vi "Plot menu activation location.vi"(8 "error in (no error)":errorcluster, 11 "MenuRef":refnum<k9>) -> (0 "error out":errorcluster, 1 "submenu tags":string[](array[string]), 2 "Location":T1, 3 "menu reference out":refnum<k9>)   [LabVIEW 2021, in "RocketPlot.lvlib"]
uses:
  RocketPlot.lvlib
  Plot menu activation submenu type.ctl
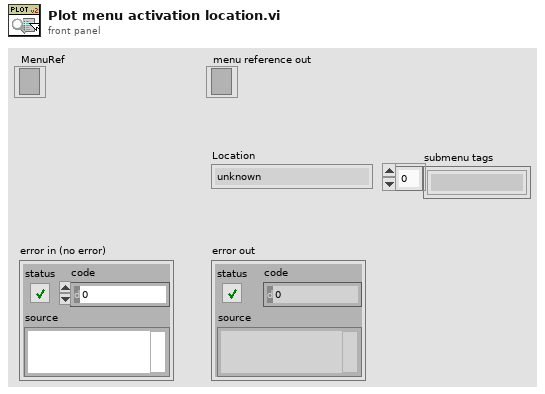
[diagram p1: front panel]
types:
  T1 = typedef "RocketPlot.lvlib/Plot menu activation submenu type.ctl" = enum16{"unknown", "plot", "legend", "x-markers", "x-scale", "y-markers", "y-scale"}
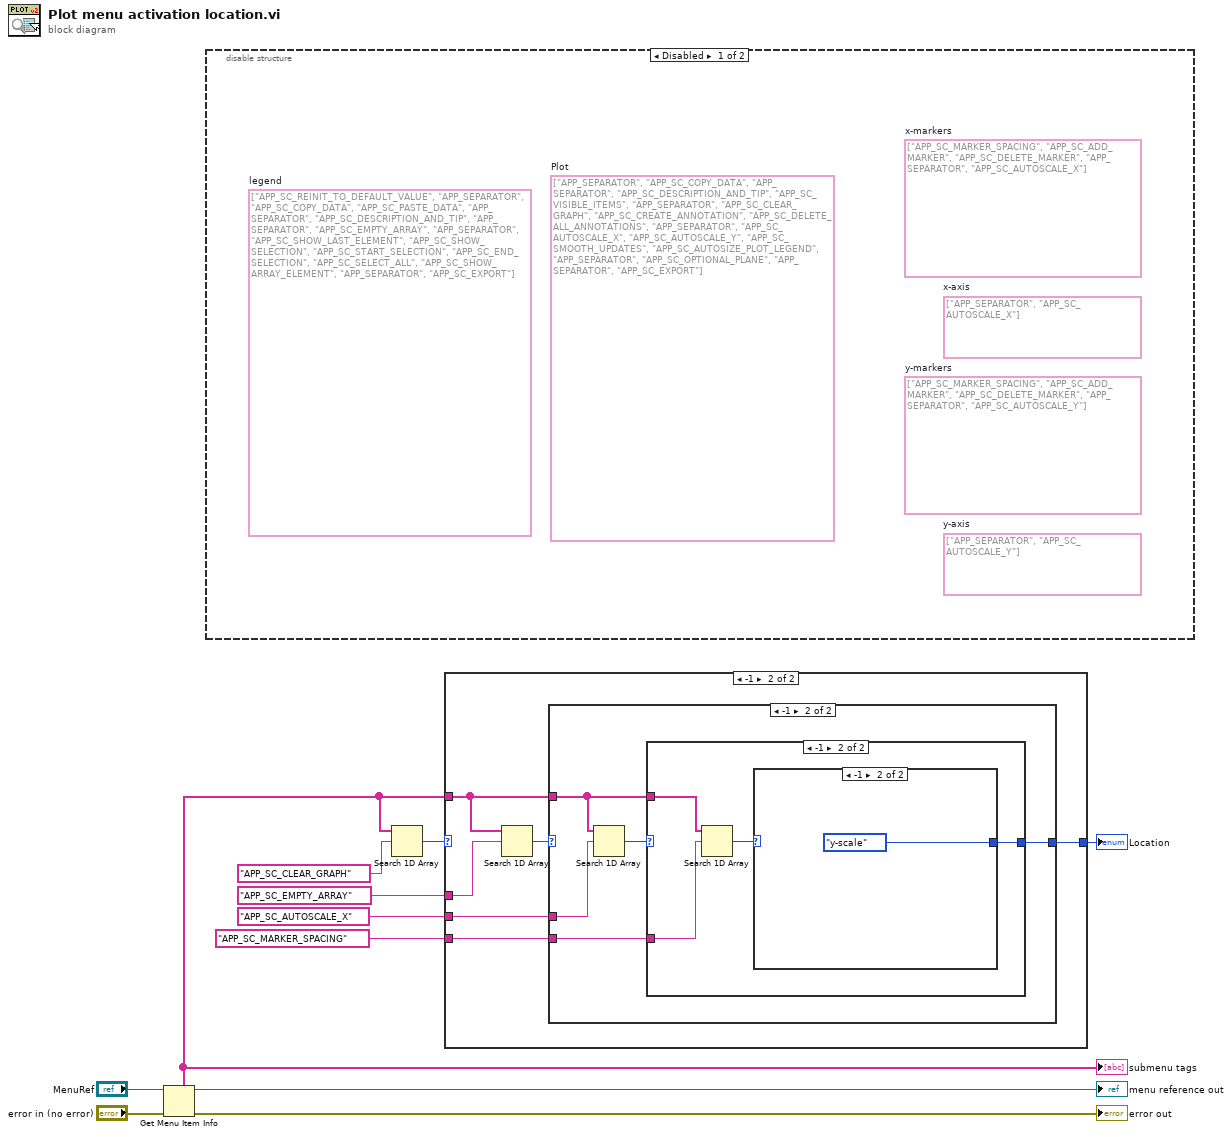
[diagram p0: block diagram]
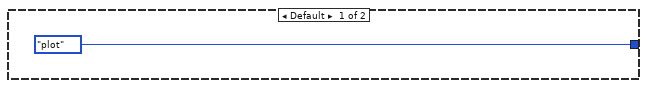
[diagram p3: hidden frame]
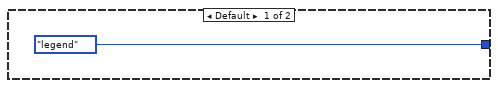
[diagram p4: hidden frame]
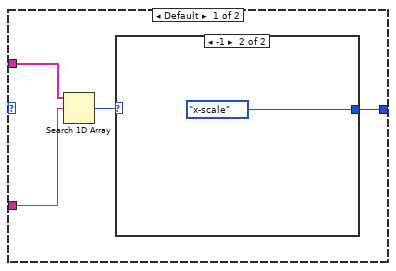
[diagram p5: hidden frame]
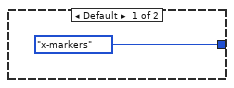
[diagram p6: hidden frame]
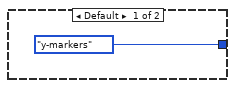
[diagram p7: hidden frame]
diagram:
  n1 = Get Menu Item Info(8:"error in (no error)", 11:"MenuRef") -> (0:→"error out":errorcluster, 3:→"menu reference out":refnum<k9>, 5:w5:string[])  [unwired: 1 in, 4 out]
  "submenu tags" <- w5
  n2 = disable-structure shown="Disabled" {
    frame Disabled {
      (unwired) string[] ["APP_SC_REINIT_TO_DEFAULT_VALUE", "APP_SEPARATOR", "APP_SC_COPY_DATA", "APP_SC_PASTE_DATA", "APP_SEPARATOR", "APP_SC_DESCRIPTION_AND_TIP", "APP_SEPARATOR", "APP_SC_EMPTY_ARRAY", "APP_SEPARATOR", "APP_SC_SHOW_LAST_ELEMENT", "APP_SC_SHOW_SELECTION", "APP_SC_START_SELECTION", "APP_SC_END_SELECTION", "APP_SC_SELECT_ALL", "APP_SC_SHOW_ARRAY_ELEMENT", "APP_SEPARATOR", "APP_SC_EXPORT"]  # legend
      (unwired) string[] ["APP_SEPARATOR", "APP_SC_COPY_DATA", "APP_SEPARATOR", "APP_SC_DESCRIPTION_AND_TIP", "APP_SC_VISIBLE_ITEMS", "APP_SEPARATOR", "APP_SC_CLEAR_GRAPH", "APP_SC_CREATE_ANNOTATION", "APP_SC_DELETE_ALL_ANNOTATIONS", "APP_SEPARATOR", "APP_SC_AUTOSCALE_X", "APP_SC_AUTOSCALE_Y", "APP_SC_SMOOTH_UPDATES", "APP_SC_AUTOSIZE_PLOT_LEGEND", "APP_SEPARATOR", "APP_SC_OPTIONAL_PLANE", "APP_SEPARATOR", "APP_SC_EXPORT"]  # Plot
      (unwired) string[] ["APP_SC_MARKER_SPACING", "APP_SC_ADD_MARKER", "APP_SC_DELETE_MARKER", "APP_SEPARATOR", "APP_SC_AUTOSCALE_X"]  # x-markers
      (unwired) string[] ["APP_SEPARATOR", "APP_SC_AUTOSCALE_X"]  # x-axis
      (unwired) string[] ["APP_SC_MARKER_SPACING", "APP_SC_ADD_MARKER", "APP_SC_DELETE_MARKER", "APP_SEPARATOR", "APP_SC_AUTOSCALE_Y"]  # y-markers
      (unwired) string[] ["APP_SEPARATOR", "APP_SC_AUTOSCALE_Y"]  # y-axis
    }
    frame Enabled {
    }
  }
  n3 = Search 1D Array(1D array=w5, element="APP_SC_CLEAR_GRAPH") -> (index of element=w9:i32)  [unwired: 1 in]
  n4 = case shown="-1" w9 {
    tunnel: w5 -> [_ w15]
    tunnel: [Plot_menu_activation_submenu_type."plot" w16] -> w3
    tunnel: "APP_SC_EMPTY_ARRAY" -> [_ w18]
    tunnel: "APP_SC_AUTOSCALE_X" -> [_ w14]
    tunnel: "APP_SC_MARKER_SPACING" -> [_ w13]
    frame Default {
    }
    frame -1 {
      n5 = Search 1D Array(1D array=w15, element=w18) -> (index of element=w17:i32)  [unwired: 1 in]
      n6 = case shown="-1" w17 {
        tunnel: [Plot_menu_activation_submenu_type."legend" w20] -> w16
        tunnel: w15 -> [_ w22]
        tunnel: w14 -> [_ w24]
        tunnel: w13 -> [_ w21]
        frame Default {
        }
        frame -1 {
          n7 = Search 1D Array(1D array=w22, element=w24) -> (index of element=w23:i32)  [unwired: 1 in]
          n8 = case shown="-1" w23 {
            tunnel: w22 -> [w28 w34]
            tunnel: w21 -> [w27 w33]
            tunnel: [w25 w31] -> w20
            frame Default {
              n9 = Search 1D Array(1D array=w28, element=w27) -> (index of element=w26:i32)  [unwired: 1 in]
              n10 = case shown="-1" w26 {
                tunnel: [Plot_menu_activation_submenu_type."x-markers" Plot_menu_activation_submenu_type."x-scale"] -> w25
                frame Default {
                }
                frame -1 {
                }
              }
            }
            frame -1 {
              n11 = Search 1D Array(1D array=w34, element=w33) -> (index of element=w32:i32)  [unwired: 1 in]
              n12 = case shown="-1" w32 {
                tunnel: [Plot_menu_activation_submenu_type."y-markers" Plot_menu_activation_submenu_type."y-scale"] -> w31
                frame Default {
                }
                frame -1 {
                }
              }
            }
          }
        }
      }
    }
  }
  "Location" <- w3
